vi "Set Multi Gate Mode [HMS].vi"(6 "Gate Number":i32, 7 "Micropulse # In":i32, 8 "error in (no error)":errorcluster, 9 "Mode":T1, 11 "Test Number":u32) -> (0 "error out":errorcluster, 5 "Micropulse # Out":i32)   [LabVIEW 2026, in "MicroPulse_Driver.lvlib"]
doc: "Multi-gate version of AMP command. The specified test is set to report amplitude and TimeBase data as follows:\n\nMode:\n= 0 First peak in gate.\n= 1 Largest peak in gate.\n= 2 All peaks reported with TimeBase.\n= 10 First Threshold crossing (single Peak).\n\nParameters:\n<Tn> : Test number. An integer value from 0 to the maximum number of tests (default maximum is 1279 tests).\nTn = 0 for all conventional tests. If the S extension is used it applies to all tests in the sweep number specified: 1-32, 0 = all sweeps.\n\n<Gn> : Gate Number, an integer value from 0 to 4.\nGn = 0 for all gates in the test\n\n<mode> : 0 1, 2 and 10\n\nSystem Compatibility: Valid in Multi-gate Mode only (AMP 31, 32 and 33)"
uses:
  MicroPulse_Driver.lvlib
  Data/Datatypes/MP - multigate mode.ctl
  Private/MP-Registry Action-Enum.ctl
  <instrlib>/Micropulse/Micropulse.lvlib
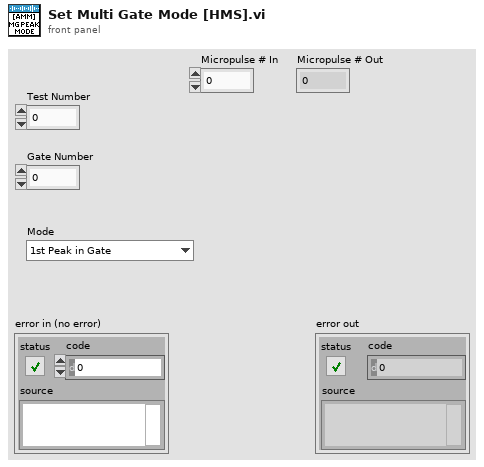
[diagram p1: front panel]
types:
  T1 = typedef "Micropulse.lvlib/MP - multigate mode.ctl" = enum16{"1st Peak in Gate", "Largest Peak In Gate", "All Peaks In Gate", "1st Threshold Crossing"}
  T2 = typedef "MicroPulse_Driver.lvlib/MP-Registry Action-Enum.ctl" = enum16{"Read", "Add Test", "Add Command", "Add Gate Command", "Add Encoder Command", "Clear Command  List", "Set Registry", "Set System Details", "Set DOF", "Set Velocity", "Disable Asynch Reads", "Enable Asynch Reads", "Add Connection", "Disconnect", "Shutdown"}
  T3 = typedef "Micropulse.lvlib/TCP config.ctl" = cluster{"Connection ID":refnum<k5>, "IP address":string, "host port":u16, "OC timeout":i32, "Read timeout":i32, "Write timeout":i32}
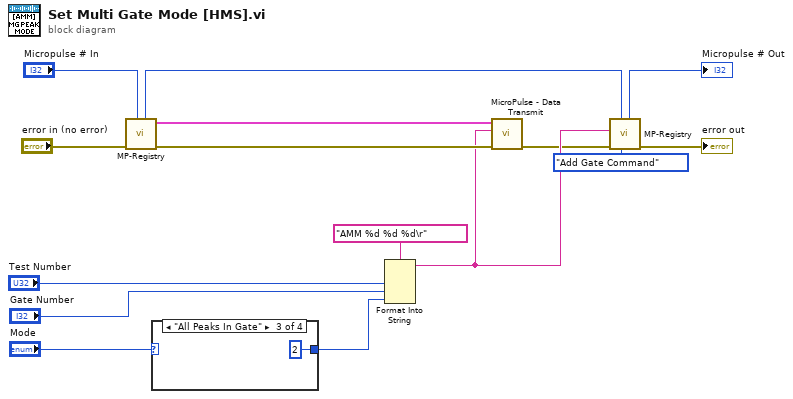
[diagram p0: block diagram]
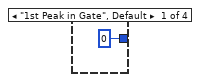
[diagram p2: hidden frame]
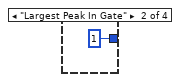
[diagram p3: hidden frame]
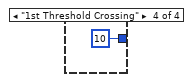
[diagram p4: hidden frame]
diagram:
  n1 = call "MP-Registry.vi"("Micropulse # In"="Micropulse # In", "error in (no error)"="error in (no error)") -> ("error out"=w13:errorcluster, "TCP config"=w12:T3, "Micropulse # Out"=w6:i32)  [unwired: 6 in, 1 out]
  n2 = case shown="\"All Peaks In Gate\"" "Mode" {
    tunnel: [0 1 2 10] -> w1
    frame "1st Peak in Gate", Default {
    }
    frame "Largest Peak In Gate" {
    }
    frame "All Peaks In Gate" {
    }
    frame "1st Threshold Crossing" {
    }
  }
  n3 = Format Into String(format string="AMM %d %d %d\r", "Test Number", "Gate Number", w1) -> (resulting string=w10:string)  [unwired: 2 in, 1 out]
  n4 = call "MicroPulse - Data Transmit.vi"("error in (no error)"=w13, "data"=w10, "TCP config"=w12) -> ("error out"=w8:errorcluster)  [unwired: 6 in, 2 out]
  n5 = call "MP-Registry.vi"("Action"=MP-Registry_Action-Enum."Add Gate Command", "Micropulse # In"=w6, "error in (no error)"=w8, "Data in"=w10) -> ("error out"=→"error out":errorcluster, "Micropulse # Out"=→"Micropulse # Out":i32)  [unwired: 4 in, 2 out]
